vi "Create Force String.vi"(11 "Channel Force Data":T1 {"Force Data" format="%x"}) -> (1 "Force info string":string, 3 "Force string":string)   [LabVIEW 2021, in "CIFLogs.lvlib"]
uses:
  CIFLogs.lvlib
  CIFCore/OOB/OOB_Rx/Typedef/Channel Fault Data.ctl
  CIFCore/OOB/OOB_Rx/CIFCoreOOB_Rx.lvclass
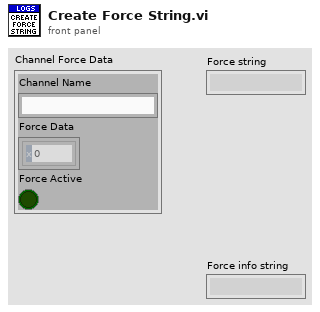
[diagram p1: front panel]
types:
  T1 = typedef "CIFCoreOOB_Rx.lvclass/Channel Fault Data.ctl" = cluster{"Channel Name":string, "Force Data":u8[], "Force Active":bool}
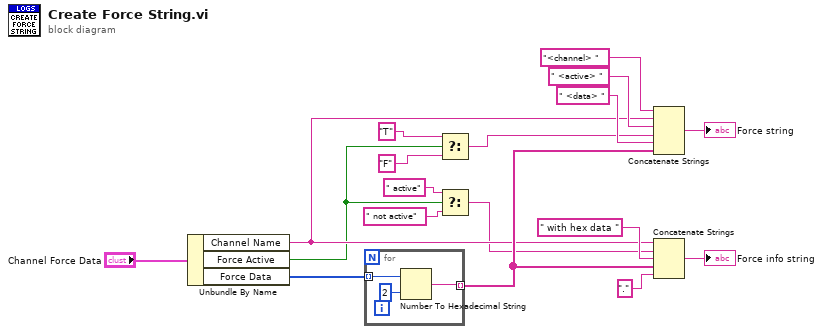
[diagram p0: block diagram]
diagram:
  n1 = Unbundle By Name("Channel Force Data") -> ("Channel Name"=w6:string, "Force Active"=w2:bool, "Force Data"=w8:u8[])
  n2 = for {
    tunnel: w8 -> [w21] mode=indexing
    tunnel: [w19] -> w7 mode=indexing
    n3 = Number To Hexadecimal String(1:i16 2 ("width (-)"), 2:w21) -> (0:w19:string)
  }
  n4 = Select(t="T" ("string"), s=w2, f="F" ("string")) -> (s? t:f=w4:string)
  n5 = Select(t=" active" ("string"), s=w2, f=" not active" ("string")) -> (s? t:f=w3:string)
  n6 = Concatenate Strings("<channel> " ("string"), w6, " <active> " ("string"), w4, " <data> " ("string"), w7) -> (→"Force string":string)
  n7 = Concatenate Strings(w6, w3, " with hex data " ("string"), w7, "." ("string")) -> (→"Force info string":string)
